vi "test_riccat_04i.vi"() -> ()   [LabVIEW 2019]
uses:
  <vilib>/Analysis/Matrix/Datatypes/RealMatrix.ctl
  <vilib>/Analysis/7linalg.llb/Real Transpose Matrix.vi
  <vilib>/Analysis/baseanly.llb/Real A x B.vi
  <vilib>/Analysis/Matrix/Numeric/Subtract/Subtract - RM,RM.vi
  <vilib>/Analysis/Matrix/Numeric/Add/Add - RM,RM.vi
  <vilib>/Analysis/baseanly.llb/Real Inverse Matrix.vi
  <vilib>/Rock Robotics/WPI/ThirdParty/JAS_Junk/TrajLib/Trajectory_Library.lvlib
  <vilib>/Analysis/NI_AALPro.lvlib
  <vilib>/Analysis/NI_AALBase.lvlib
  <vilib>/Analysis/Matrix/NI_Matrix.lvlib
panel:
  out "Finished":bool
  out "Iterations":i32
  out "Elapsed \nTime MS":dbl
  out "Err 4":i32
  out "Err 3":i32
  out "Err 2":i32
  out "Err 1":i32
  out "Err 9":i32
  out "ZERO":T1
  out "X  Answer":T1
  in  "R":T1=[[1.0, 0.0], [0.0, 1.0]]
  in  "Q":T1=[[1.0, 0.0], [0.0, 1.0]]
  in  "B":T1=[[1.0], [0.0], [0.0], [1.0]]
  in  "A":T1=[[1.0, 0.0], [0.0, 1.0]]
  # "// ------------------------------------------------------------\n  // Test 4: A = B = Q = R = I_2 (2-by-2 identity matrix)"
  # "A4 << \n           1, 0, \n            0, 1;"
  # "B4 << \n    1, \n    0, \n    0, \n    1;"
  # "Solution weight ??"
  # "Q4 << \n        1, 0, \n         0, 1;"
  # "Cost ??"
  # "R4 << \n        1, 0, \n        0, 1;"
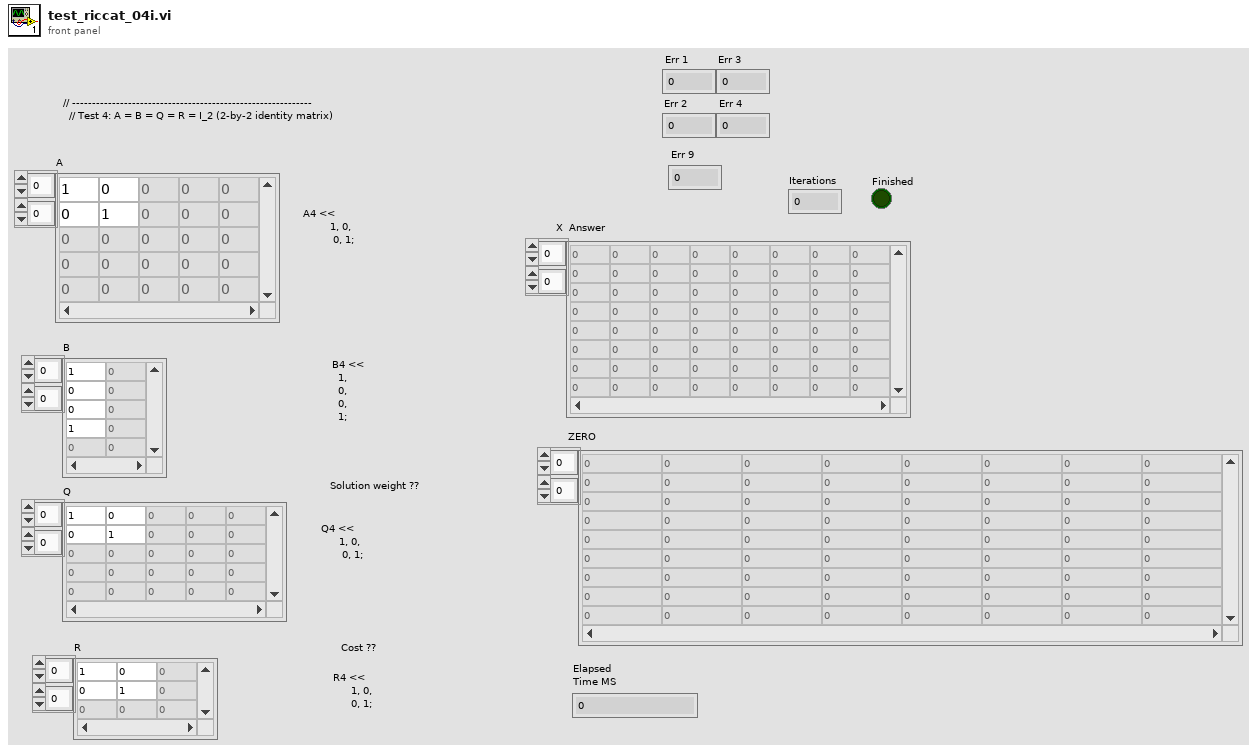
[diagram p1: front panel]
types:
  T1 = typedef "NI_Matrix.lvlib/RealMatrix.ctl" = dbl[][]
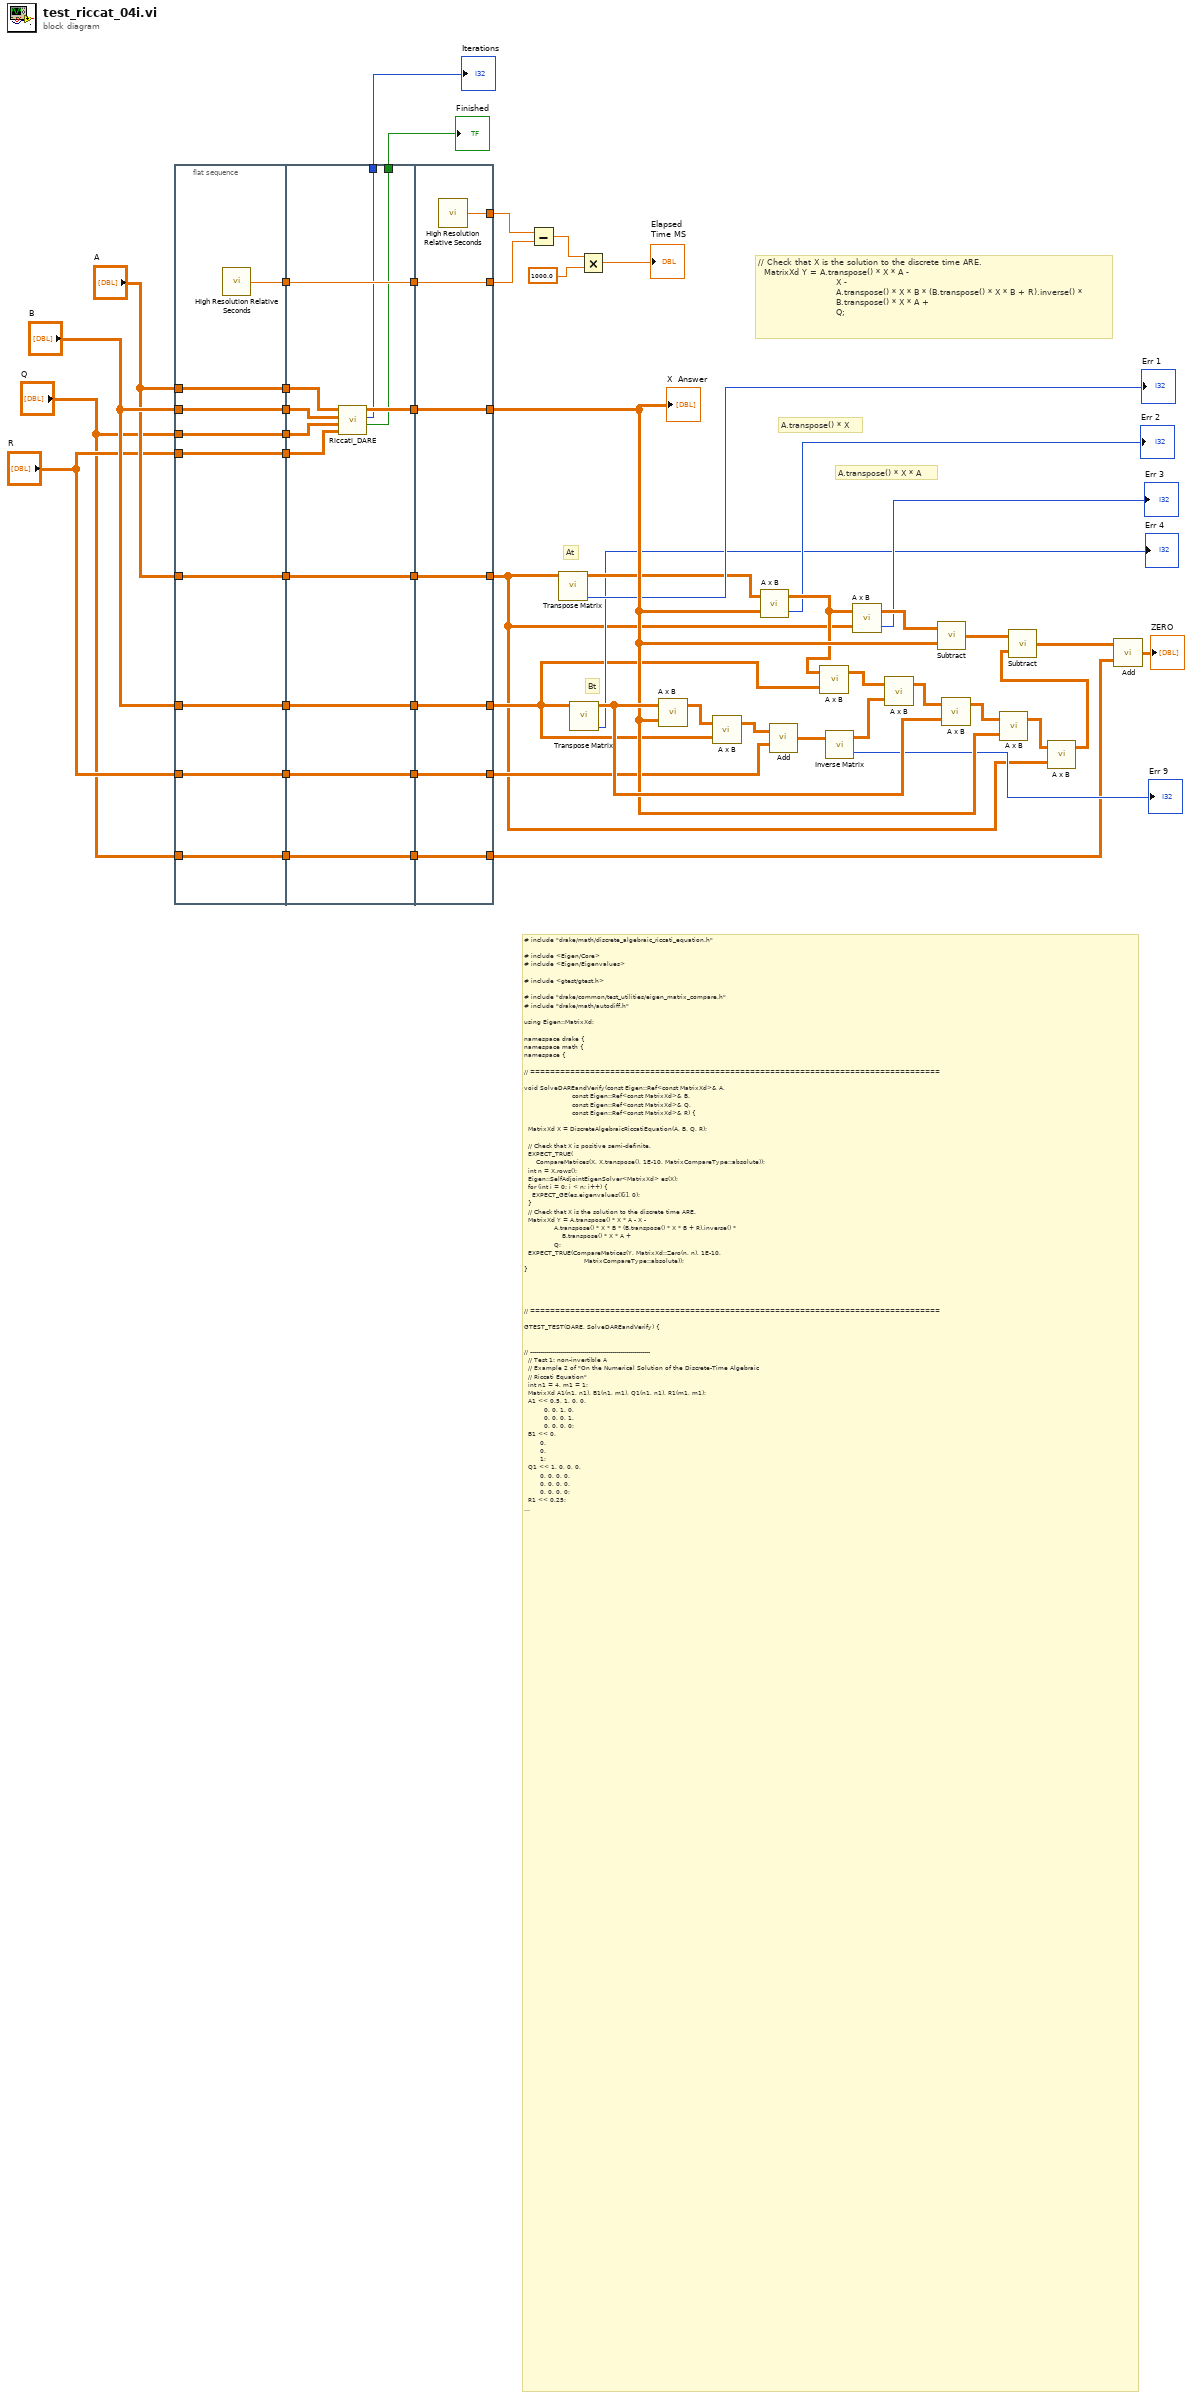
[diagram p0: block diagram]
diagram:
  # "A.transpose() * X"
  # "A.transpose() * X * A"
  # "Bt"
  # "At"
  # "// Check that X is the solution to the discrete time ARE.\n  MatrixXd Y = A.transpose() * X * A - \n                          X -\n                          A.transpose() * X * B * (B.transpose() * X * B + R).inverse() *\n                          B.transpose() * X * A +\n                          Q;"
  # "# include \"drake/math/discrete_algebraic_riccati_equation.h\"\n\n# include <Eigen/Core>\n# include <Eigen/Eigenvalues>\n\n# include <gtest/gtest.h>\n\n# include \"drake/common/test_utilities/eigen_matrix_compare.h\"\n# include \"drake/math/autodiff.h\"\n\nusing Eigen::MatrixXd;\n\nnamespace drake {\nnamespace math {\nnamespace {\n\n// ==================================================================================\n\nvoid SolveDAREandVerify(const Eigen::Ref<const MatrixXd>& A,\n                        const Eigen::Ref<const MatrixXd>& B,\n                        const Eigen::Ref<const MatrixXd>& Q,\n                        const Eigen::Ref<const MatrixXd>& R) {\n\n  MatrixXd X = DiscreteAlgebraicRiccatiEquation(A, B, Q, R);\n\n  // Check that X is positive semi-definite.\n  EXPECT_TRUE(\n      CompareMatrices(X, X.transpose(), 1E-10, MatrixCompareType::absolute));\n  int n = X.rows();\n  Eigen::SelfAdjointEigenSolver<MatrixXd> es(X);\n  for (int i = 0; i < n; i++) {\n    EXPECT_GE(es.eigenvalues()[i], 0);\n  }\n  // Check that X is the solution to the discrete time ARE.\n  MatrixXd Y = A.transpose() * X * A - X -\n               A.transpose() * X * B * (B.transpose() * X * B + R).inverse() *\n                   B.transpose() * X * A +\n               Q;\n  EXPECT_TRUE(CompareMatrices(Y, MatrixXd::Zero(n, n), 1E-10,\n                              MatrixCompareType::absolute));\n}\n\n\n\n\n// ==================================================================================\n\nGTEST_TEST(DARE, SolveDAREandVerify) {\n\n\n// ------------------------------------------------------------\n  // Test 1: non-invertible A\n  // Example 2 of \"On the Numerical Solution of the Discrete-Time Algebraic\n  // Riccati Equation\"\n  int n1 = 4, m1 = 1;\n  MatrixXd A1(n1, n1), B1(n1, m1), Q1(n1, n1), R1(m1, m1);\n  A1 << 0.5, 1, 0, 0, \n          0, 0, 1, 0, \n          0, 0, 0, 1, \n          0, 0, 0, 0;\n  B1 << 0, \n        0, \n        0, \n        1;\n  Q1 << 1, 0, 0, 0, \n        0, 0, 0, 0, \n        0, 0, 0, 0, \n        0, 0, 0, 0;\n  R1 << 0.25;\n  SolveDAREandVerify(A1, B1, Q1, R1);\n// ------------------------------------------------------------\n  // Test 2: invertible A\n  int n2 = 2, m2 = 1;\n  MatrixXd A2(n2, n2), B2(n2, m2), Q2(n2, n2), R2(m2, m2);\n  A2 << 1, 1, 0, 1;\n  B2 << 0, 1;\n  Q2 << 1, 0, 0, 0;\n  R2 << 0.3;\n  SolveDAREandVerify(A2, B2, Q2, R2);\n\n// ------------------------------------------------------------\n  // Test 3: the first generalized eigenvalue of (S,T) is stable\n  int n3 = 2, m3 = 1;\n  MatrixXd A3(n3, n3), B3(n3, m3), Q3(n3, n3), R3(m3, m3);\n  A3 << 0, 1, 0, 0;\n  B3 << 0, 1;\n  Q3 << 1, 0, 0, 1;\n  R3 << 1;\n  SolveDAREandVerify(A3, B3, Q3, R3);\n\n// ------------------------------------------------------------\n  // Test 4: A = B = Q = R = I_2 (2-by-2 identity matrix)\n  int n4 = 2, m4 = 2;\n  MatrixXd A4(n4, n4), B4(n4, m4), Q4(n4, n4), R4(m4, m4);\n  A4 << 1, 0, 0, 1;\n  B4 << 1, 0, 0, 1;\n  Q4 << 1, 0, 0, 1;\n  R4 << 1, 0, 0, 1;\n  SolveDAREandVerify(A4, B4, Q4, R4);\n\n// ------------------------------------------------------------\n}\n}  // namespace\n}  // namespace math\n}  // namespace drake"
  n1 = flat-sequence {
    tunnel: "B" -> [w56]
    tunnel: "A" -> [w57]
    tunnel: "B" -> [w58]
    tunnel: "Q" -> [w59]
    tunnel: "A" -> [w60]
    tunnel: "R" -> [w61]
    tunnel: [w61] -> w30
    tunnel: [w60] -> w29
    tunnel: [w59] -> w28
    tunnel: [w58] -> w27
    tunnel: [w57] -> w26
    tunnel: [w56] -> w25
    tunnel: "R" -> [w55]
    tunnel: [w55] -> w17
    tunnel: "Q" -> [w54]
    tunnel: [w54] -> w14
    tunnel: [w53] -> w7
    tunnel: w30 -> [w73]
    tunnel: w29 -> [w71]
    tunnel: w28 -> [w70]
    tunnel: w27 -> [w69]
    tunnel: w26 -> [w68]
    tunnel: w25 -> [w67]
    tunnel: [w72] -> w24
    tunnel: [w68] -> w23
    tunnel: [w67] -> w22
    tunnel: [w66] -> w18
    tunnel: w17 -> [w66]
    tunnel: w14 -> [w65]
    tunnel: [w65] -> w13
    tunnel: [w64] -> w8
    tunnel: w7 -> [w64]
    tunnel: [w63] -> w3
    tunnel: [w62] -> w2
    tunnel: [w78] -> w20
    tunnel: [w79] -> w1
    tunnel: [w80] -> w44
    tunnel: w24 -> [w80]
    tunnel: w23 -> [w79]
    tunnel: w22 -> [w78]
    tunnel: [w77] -> w15
    tunnel: w18 -> [w77]
    tunnel: [w76] -> w11
    tunnel: w13 -> [w76]
    tunnel: [w75] -> w10
    tunnel: [w74] -> w9
    tunnel: w8 -> [w74]
    frame #0 {
      n2 = call <vilib>:"High Resolution Relative Seconds.vi"() -> ("relative seconds"=w53:dbl)
    }
    frame #1 {
      n3 = call <vilib>:"Riccati_DARE.vi"("R"=w73, "Q"=w70, "B"=w69, "A"=w71) -> ("Error"=w62:bool, "Iterations"=w63:i32, "Answer"=w72:T1)  [unwired: 5 in]
    }
    frame #2 {
      n4 = call <vilib>:"High Resolution Relative Seconds.vi"() -> ("relative seconds"=w75:dbl)
    }
  }
  n5 = Subtract(x=w10, y=w9) -> (x-y=w6:dbl)
  n6 = call-poly <vilib>:"Transpose Matrix.vi"("Input Matrix"=w1) -> ("error"=→"Err 1":i32, "Matrix Transpose"=w34:T1)  [unwired: 9 in]
  n7 = call-poly <vilib>:"Transpose Matrix.vi"("Input Matrix"=w20) -> ("error"=→"Err 4":i32, "Matrix Transpose"=w46:T1)  [unwired: 9 in]
  n8 = Multiply(x=w6, y=1000.0) -> (x*y=→"Elapsed \nTime MS":dbl)
  n9 = call-poly <vilib>:"A x B.vi"("B"=w44, "A"=w46) -> ("A x B"=w51:T1)  [unwired: 1 out]
  n10 = call-poly <vilib>:"A x B.vi"("B"=w20, "A"=w51) -> ("A x B"=w50:T1)  [unwired: 1 out]
  n11 = call-poly <vilib>:"A x B.vi"("B"=w44, "A"=w34) -> ("error"=→"Err 2":i32, "A x B"=w37:T1)
  n12 = call-poly <vilib>:"Add.vi"("Real Matrix B"=w15, "Real Matrix A"=w50) -> ("A + B"=w49:T1)
  n13 = call-poly <vilib>:"A x B.vi"("B"=w20, "A"=w37) -> ("A x B"=w36:T1)  [unwired: 1 out]
  n14 = call-poly <vilib>:"Inverse Matrix.vi"("Input Matrix"=w49) -> ("error"=→"Err 9":i32, "Inverse Matrix"=w48:T1)  [unwired: 1 in]
  n15 = call-poly <vilib>:"A x B.vi"("B"=w1, "A"=w37) -> ("error"=→"Err 3":i32, "A x B"=w52:T1)
  n16 = call-poly <vilib>:"A x B.vi"("B"=w48, "A"=w36) -> ("A x B"=w47:T1)  [unwired: 1 out]
  n17 = call-poly <vilib>:"Subtract.vi"("Real Matrix B"=w44, "Real Matrix A"=w52) -> ("A - B"=w42:T1)
  n18 = call-poly <vilib>:"A x B.vi"("B"=w46, "A"=w47) -> ("A x B"=w45:T1)  [unwired: 1 out]
  n19 = call-poly <vilib>:"A x B.vi"("B"=w44, "A"=w45) -> ("A x B"=w43:T1)  [unwired: 1 out]
  n20 = call-poly <vilib>:"A x B.vi"("B"=w1, "A"=w43) -> ("A x B"=w41:T1)  [unwired: 1 out]
  n21 = call-poly <vilib>:"Subtract.vi"("Real Matrix B"=w41, "Real Matrix A"=w42) -> ("A - B"=w40:T1)
  n22 = call-poly <vilib>:"Add.vi"("Real Matrix B"=w11, "Real Matrix A"=w40) -> ("A + B"=→"ZERO":T1)
  "X  Answer" <- w44
  "Iterations" <- w3
  "Finished" <- w2
